vi "CTS_GetWaveform.vi"(3 "Stop Wvl":dbl=1570.0 format="%.3f", 4 "StartWvl":dbl=1520.0 format="%.3f", 5 "address string":string="25") -> (1 "Output Array":cluster{dbl[], dbl[]}(graph))   [LabVIEW 2009]
uses:
  <vilib>/Utility/file.llb/Write To Spreadsheet File (DBL).vi
panel:
  out "x/y":dbl format="%.6f"
  out "Numeric 3":dbl format="%.4f"
  out "Numeric 2":i32
  out "Numeric":dbl format="%.4f"
  in  "Save Data?":bool
  in  "stop":bool=TRUE
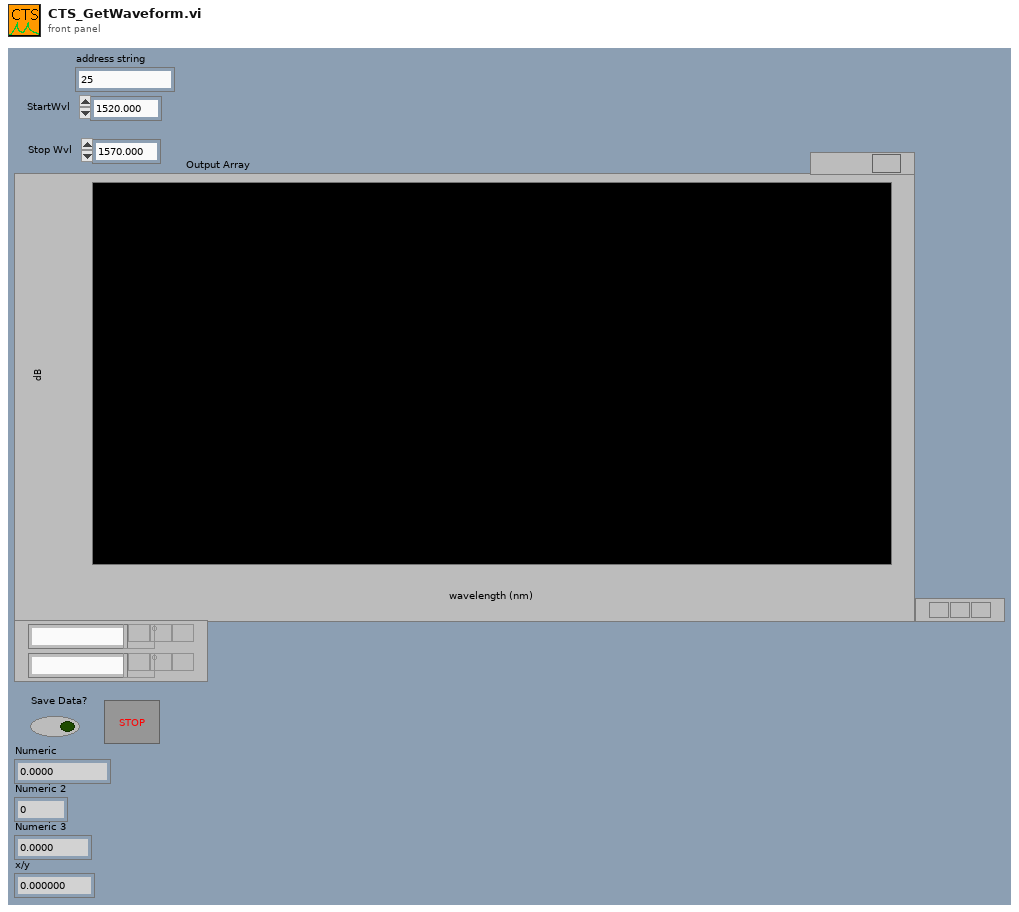
[diagram p1: front panel]
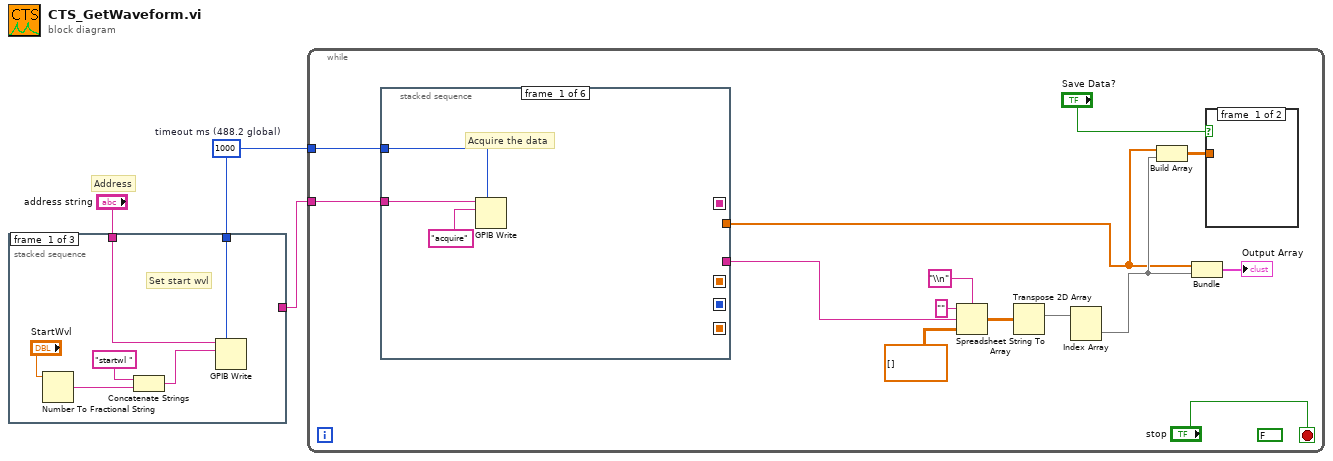
[diagram p0: block diagram]
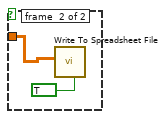
[diagram p2: hidden frame]
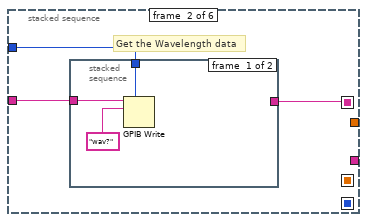
[diagram p3: hidden frame]
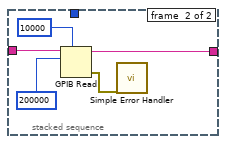
[diagram p4: hidden frame]
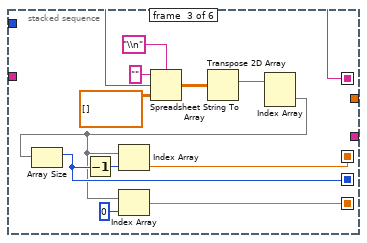
[diagram p5: hidden frame]
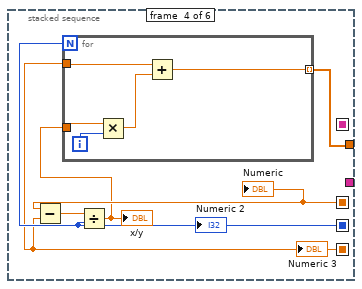
[diagram p6: hidden frame]
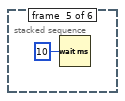
[diagram p7: hidden frame]
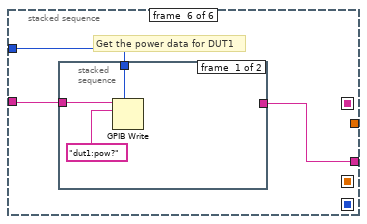
[diagram p8: hidden frame]
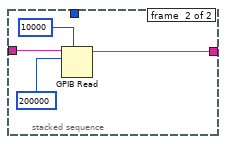
[diagram p9: hidden frame]
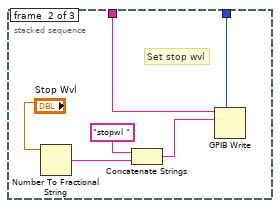
[diagram p10: hidden frame]
diagram:
  w1 = 1000  # timeout ms (488.2 global)
  # "Address"
  n1 = stacked-sequence {
    tunnel: "address string" -> [w9 w15 w16]
    tunnel: [_ _ w16] -> w2
    tunnel: w1 -> [w8 w14 _]
    frame #0 {
      # "Set start wvl"
      n2 = Number To Fractional String(number="StartWvl") -> (F-format string=w4:string)  [unwired: 3 in]
      n3 = Concatenate Strings("startwl " ("data"), w4) -> (w6:string)
      n4 = GPIB Write(0:w9, 1:w6, 4:w8) -> ()  [unwired: 2 in, 2 out]
    }
    frame #1 {
      # "Set stop wvl"
      n5 = Number To Fractional String(number="Stop Wvl") -> (F-format string=w13:string)  [unwired: 3 in]
      n6 = Concatenate Strings("stopwl " ("data"), w13) -> (w10:string)
      n7 = GPIB Write(0:w15, 1:w10, 4:w14) -> ()  [unwired: 2 in, 2 out]
    }
    frame #2 {
    }
  }
  n8 = while {
    tunnel: w1 -> [w22]
    tunnel: w2 -> [w30]
    stop <- "stop" stop-if-true
    (unwired) FALSE
    n9 = stacked-sequence {
      seq-local: [_ w36 _ _ _ _] -> [_ _ w53 _ _ _]
      seq-local: [_ _ w51 _ _ _] -> [_ _ _ w64 _ _]
      seq-local: [_ _ w50 _ _ _] -> [_ _ _ w61 _ _]
      seq-local: [_ _ w49 _ _ _] -> [_ _ _ w62 _ _]
      tunnel: w30 -> [w35 w38 _ _ _ w73]
      tunnel: [_ _ _ _ _ w72] -> w29
      tunnel: w22 -> [w33 w37 _ _ _ w71]
      tunnel: [_ _ _ w59 _ _] -> w17
      frame #0 {
        # "Acquire the data"
        n10 = GPIB Write(0:w35, 1:"acquire" ("data"), 4:w33) -> ()  [unwired: 2 in, 2 out]
      }
      frame #1 {
        # "Get the Wavelength data"
        n11 = stacked-sequence {
          tunnel: w38 -> [w41 w46]
          tunnel: [_ w45] -> w36
          tunnel: w37 -> [w39 _]
          frame #0 {
            n12 = GPIB Write(0:w41, 1:"wav?" ("data"), 4:w39) -> ()  [unwired: 2 in, 2 out]
          }
          frame #1 {
            n13 = GPIB Read(0:w46, 1:200000 ("byte count"), 4:10000 ("timeout ms (488.2 global)")) -> (5:w45:string, 7:w43:errorcluster)  [unwired: 2 in, 1 out]
            n14 = call <vilib>:"Simple Error Handler.vi"("error in (no error)"=w43) -> ()  [unwired: 4 in, 5 out]
          }
        }
      }
      frame #2 {
        n15 = Spreadsheet String To Array(delimiter (Tab)="\\n", format string="", spreadsheet string=w53, array type (2D Dbl)=dbl[][] []) -> (array=w57:dbl[][])
        n16 = Transpose 2D Array(2D array=w57) -> (transposed array=w58:dbl[][])
        n17 = Index Array(array=w58) -> (element=w47:dbl[])  [unwired: 2 in]
        n18 = Array Size(array=w47) -> (size(s)=w49:i32)
        n19 = Decrement(x=w49) -> (x-1=w48:i32)
        n20 = Index Array(array=w47, index=w48) -> (element=w51:dbl)
        n21 = Index Array(array=w47, index=0 ("Index")) -> (element=w50:dbl)
      }
      frame #3 {
        n22 = Subtract(x=w64, y=w61) -> (x-y=w63:dbl)
        n23 = Divide(x=w63, y=w62) -> (x/y=w60:dbl)
        "x/y" <- w60
        n24 = for {
          N: w62 -> [_]
          tunnel: w61 -> [w67]
          tunnel: w60 -> [w68]
          tunnel: [w65] -> w59 mode=indexing
          i -> [w69]
          n25 = Multiply(x=w68, y=w69) -> (x*y=w66:dbl)
          n26 = Add(x=w67, y=w66) -> (x+y=w65:dbl)
        }
        "Numeric" <- w64
        "Numeric 2" <- w62
        "Numeric 3" <- w61
      }
      frame #4 {
        n27 = Wait (ms)(milliseconds to wait=u32 10) -> ()  [unwired: 1 out]
      }
      frame #5 {
        # "Get the power data for DUT1"
        n28 = stacked-sequence {
          tunnel: w73 -> [w76 w80]
          tunnel: [_ w79] -> w72
          tunnel: w71 -> [w74 _]
          frame #0 {
            n29 = GPIB Write(0:w76, 1:"dut1:pow?" ("data"), 4:w74) -> ()  [unwired: 2 in, 2 out]
          }
          frame #1 {
            n30 = GPIB Read(0:w80, 1:200000 ("byte count"), 4:10000 ("timeout ms (488.2 global)")) -> (5:w79:string)  [unwired: 2 in, 2 out]
          }
        }
      }
    }
    n31 = Spreadsheet String To Array(delimiter (Tab)="\\n", format string="", spreadsheet string=w29, array type (2D Dbl)=dbl[][] []) -> (array=w25:dbl[][])
    n32 = Transpose 2D Array(2D array=w25) -> (transposed array=w24:dbl[][])
    n33 = Index Array(array=w24) -> (element=w21:dbl[])  [unwired: 2 in]
    n34 = Build Array(w17, w21) -> (w20:dbl[][])
    n35 = Bundle(w17, w21) -> (→"Output Array":cluster{dbl[], dbl[]})  [unwired: 1 in]
    n36 = case shown="True" "Save Data?" {
      tunnel: w20 -> [_ w32]
      frame #0 {
      }
      frame #1 {
        n37 = call-poly <vilib>:"Write To Spreadsheet File.vi"("transpose? (no:F)"=TRUE, "2D data"=w32) -> ()  [unwired: 6 in, 1 out]
      }
    }
  }
